vi "Get Worksheet.Ref.vi"(8 "error in (no error)":errorcluster, 11 "worksheet in":refnum<class "worksheet.lvclass">) -> (0 "error out":errorcluster, 2 "Worksheet.Ref":refnum<k24>, 3 "worksheet out":refnum<class "worksheet.lvclass">)   [LabVIEW 2017, in "Excel_Specific.lvlib" / "worksheet.lvclass"]
uses:
  worksheet.lvclass
  C:/Users/Neo/Desktop/Dev_Tools_BR/LabVIEW_NPOI/src/lib/NPOI 2.1.1/NPOI.dll
  lib/NPOI 2.1.1/NPOI.dll
  worksheet.lvclass/worksheet.ctl
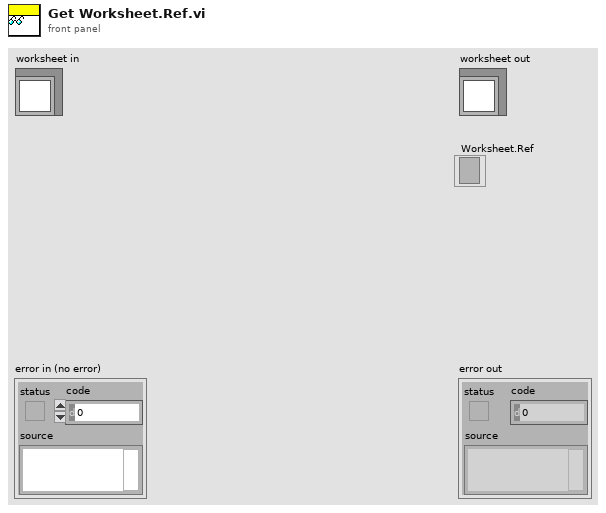
[diagram p1: front panel]
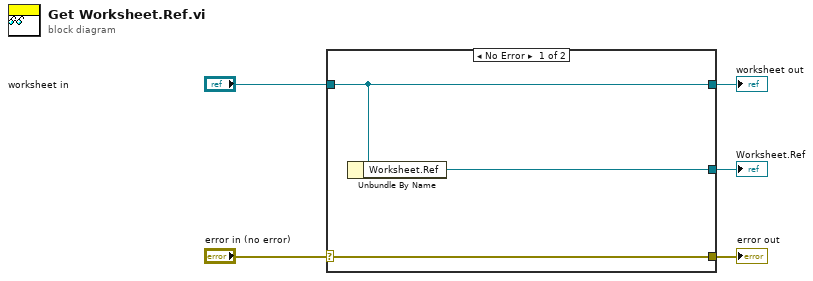
[diagram p0: block diagram]
diagram:
  n1 = case shown="No Error" "error in (no error)" {
    selector: "error in (no error)" -> [w8 w9]
    tunnel: [w8 w9] -> w4
    tunnel: [w7 w10] -> w2
    tunnel: "worksheet in" -> [w7 w10]
    tunnel: [w6 _] -> w1
    frame No Error {
      n2 = Unbundle By Name(w7) -> ("Worksheet.Ref"=w6:refnum<k24>)
    }
    frame Error {
    }
  }
  "error out" <- w4
  "worksheet out" <- w2
  "Worksheet.Ref" <- w1
